vi "Get_VI_front_panel_scaling_setting.vi"(0 "reference":refnum<vi>, 1 "error in (no error)":errorcluster) -> (2 "reference out":refnum<vi>, 3 "scaling":T1 items=["Unchanged", "No Scaling", "Scale front panel to fit"], 4 "error out":errorcluster)   [LabVIEW 2017, in "NI_ReportGenerationCore.lvlib"]
uses:
  <vilib>/Utility/NIReport.llb/NI_ReportGenerationCore.lvlib
  <vilib>/printing/EasyPrintingControls.llb/panel_scaling_for_page.ctl
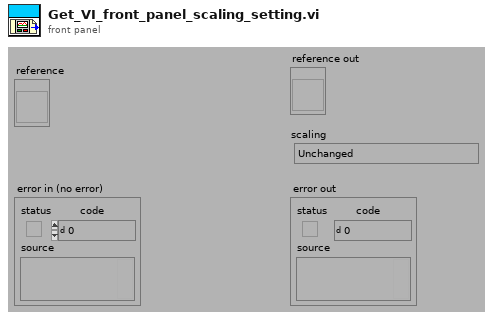
[diagram p1: front panel]
types:
  T1 = typedef "NI_ReportGenerationCore.lvlib/panel_scaling_for_page.ctl" = u16
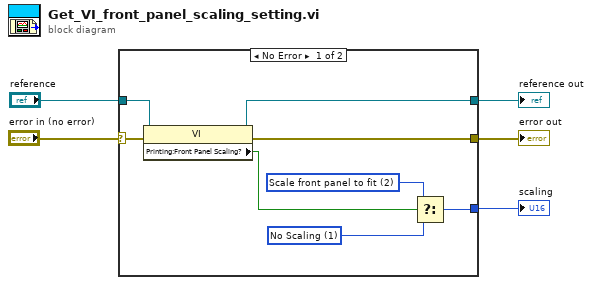
[diagram p0: block diagram]
diagram:
  n1 = case shown="No Error" "error in (no error)" {
    selector: "error in (no error)" -> [w12 w15]
    tunnel: [w8 w14] -> w5
    tunnel: [w11 w15] -> w4
    tunnel: "reference" -> [w9 w14]
    tunnel: [w6 _] -> w1
    frame No Error {
      w10 = T1 1 items=["Unchanged", "No Scaling", "Scale front panel to fit"] ("panel scaling for page (unchanged)")
      w7 = T1 2 items=["Unchanged", "No Scaling", "Scale front panel to fit"] ("panel scaling for page (unchanged)")
      n2 = property class="VI"(reference=w9, error in=w12) -> (reference out=w8:refnum<vi>, error out=w11:errorcluster, "Printing:Front Panel Scaling?"=w13:bool)
      n3 = Select(t=w7, s=w13, f=w10) -> (s? t:f=w6:T1)
    }
    frame Error {
    }
  }
  "reference out" <- w5
  "error out" <- w4
  "scaling" <- w1
